vi "Generic Request (Buffer).vi"(5 "method":string, 6 "timeout":i32=10000, 7 "output file":path, 8 "error in":errorcluster, 9 "buffer":string, 10 "url":string, 11 "session in":refnum<class "Session.lvclass">) -> (0 "error out":errorcluster, 1 "body":string, 2 "headers":string, 3 "session out":refnum<class "Session.lvclass">, 4 "status code":u32)   [LabVIEW 2024, in "lib_NI_Advanced HTTP Client.lvlib" / "Session.lvclass"]
uses:
  Session.lvclass
  Session.lvclass/Session.ctl
  lvwebclient_64.dll
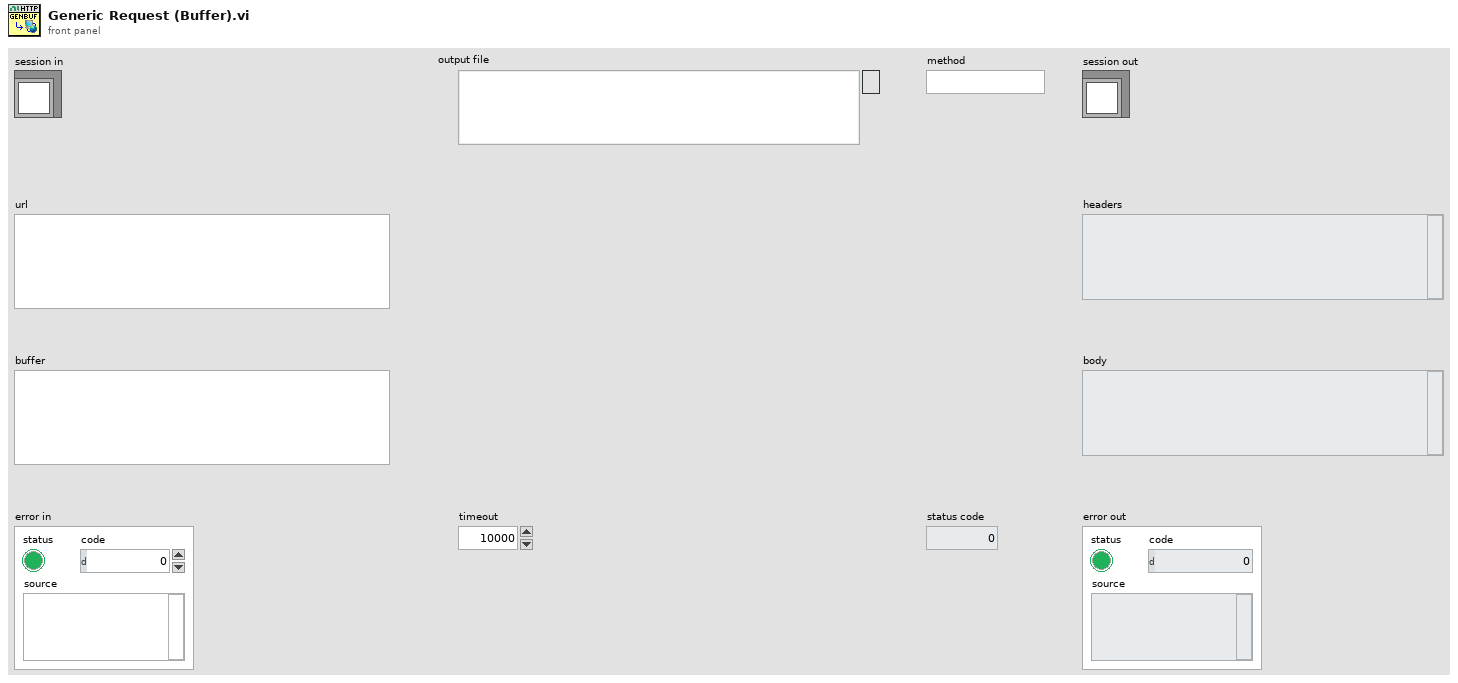
[diagram p1: front panel]
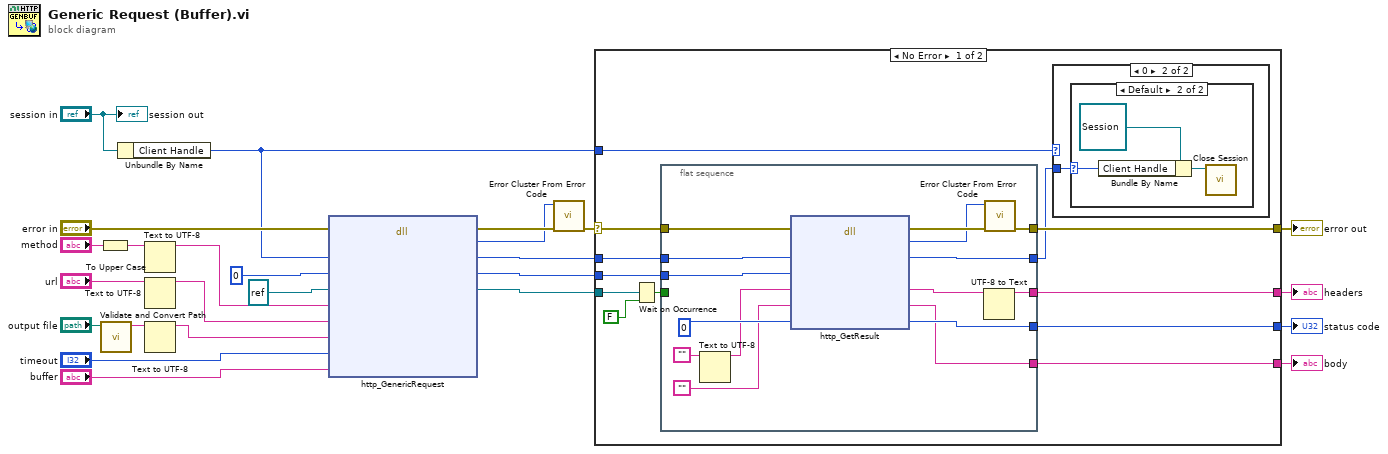
[diagram p0: block diagram]
diagram:
  n1 = To Upper Case(1:"method") -> (0:w1:string)
  n2 = call "Validate and Convert Path.vi"("path"="output file") -> ("validated path as string"=w17:string)  [unwired: 10 in]
  n3 = Unbundle By Name("session in") -> ("Client Handle"=w7:u32)
  n4 = Text to UTF-8(11:w1) -> (3:w3:string)  [unwired: 2 in, 1 out]
  n5 = Text to UTF-8(11:"url") -> (3:w6:string)  [unwired: 2 in, 1 out]
  n6 = Text to UTF-8(11:w17) -> (3:w5:string)  [unwired: 2 in, 1 out]
  n7 = dll-call lib="C:/Program Files/National Instruments/LabVIEW 2024/vi.lib/NI/Advanced HTTP Client/lvwebclient_*.*" fn="http_GenericRequest"(error in="error in", "handle"=w7, "request"=u32 0, "completeOccurrence"=refnum<k4> refnum ("occurrence"), "method"=w3, "url"=w6, "outPath"=w5, "timeoutInMs"="timeout", "requestBody"="buffer") -> (error out=w15:errorcluster, "return"=w14:i32, "handle"=w13:u32, "request"=w12:u32, "completeOccurrence"=w10:refnum<k4>)  [unwired: 7 in, 1 out]
  n8 = call "Error Cluster From Error Code.vi"("error in (no error)"=w15, "error code (0)"=w14) -> ("error out"=w25:errorcluster)  [unwired: 7 in]
  n9 = case shown="No Error" w25 {
    selector: w25 -> [w35 w57]
    tunnel: w10 -> [w37 _]
    tunnel: w13 -> [w34 _]
    tunnel: w12 -> [w33 _]
    tunnel: [w32 _] -> w22
    tunnel: [w31 _] -> w21
    tunnel: [w30 _] -> w20
    tunnel: [w29 w57] -> w19
    tunnel: w7 -> [w28 _]
    frame No Error {
      n10 = Wait on Occurrence(1:FALSE, 2:w37) -> (0:w36:bool)  [unwired: 1 in]
      n11 = flat-sequence {
        tunnel: w36 -> [_]
        tunnel: w35 -> [w56]
        tunnel: w34 -> [w55]
        tunnel: w33 -> [w54]
        tunnel: [w52] -> w32
        tunnel: [w47] -> w31
        tunnel: [w48] -> w30
        tunnel: [w46] -> w29
        tunnel: [w45] -> w27
        frame #0 {
          n12 = Text to UTF-8(11:"") -> (3:w43:string)  [unwired: 2 in, 1 out]
          n13 = dll-call lib="C:/Program Files/National Instruments/LabVIEW 2024/vi.lib/NI/Advanced HTTP Client/lvwebclient_*.*" fn="http_GetResult"(error in=w56, "handle"=w55, "request"=w54, "returnHeader"=w43, "returnBody"="", "httpStatus"=u32 0) -> (error out=w51:errorcluster, "return"=w50:i32, "handle"=w45:u32, "returnHeader"=w49:string, "returnBody"=w48:string, "httpStatus"=w52:u32)  [unwired: 3 in, 1 out]
          n14 = UTF-8 to Text(11:w49) -> (3:w47:string)  [unwired: 2 in, 1 out]
          n15 = call "Error Cluster From Error Code.vi"("error in (no error)"=w51, "error code (0)"=w50) -> ("error out"=w46:errorcluster)  [unwired: 7 in]
        }
      }
      n16 = case shown="0" w28 {
        tunnel: w27 -> [_ w38]
        frame Default {
        }
        frame 0 {
          n17 = case shown="Default" w38 {
            selector: w38 -> [_ w41]
            frame 0 {
            }
            frame Default {
              n18 = Bundle By Name(cluster=refnum<class "Session.lvclass"> refnum ("NI_Advanced HTTP Client.lvlib:Session.lvclass"), "Client Handle"=w41) -> (w40:refnum<class "Session.lvclass">)
              n19 = call "Close Session.vi"("session"=w40) -> ()  [unwired: 10 in, 1 out]
            }
          }
        }
      }
    }
    frame Error {
    }
  }
  "error out" <- w19
  "headers" <- w21
  "body" <- w20
  "status code" <- w22
  "session out" <- "session in"
